vi "GetSpectrum_Fast_sub.vi"() -> (0 "array":i32[](array[numeric]), 1 "from GetStatus 2":T1, 2 "from Get Acq Data":u32, 3 "from Start Acq":u32)   [LabVIEW 2021]
uses:
  <userlib>/atmcd32d.llb/Error Code Enum typedef.ctl
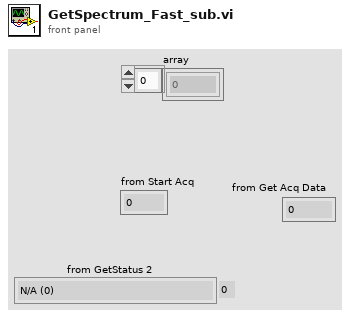
[diagram p1: front panel]
types:
  T1 = typedef "Error Code Enum typedef.ctl" = enum32{"N/A (0)", "DRV_ERROR_CODES", "DRV_SUCCESS", "DRV_VXDNOTINSTALLED", "DRV_ERROR_SCAN", "DRV_ERROR_CHECK_SUM", "DRV_ERROR_FILELOAD", "DRV_UNKNOWN_FUNC", "DRV_ERROR_VXD_INIT", "DRV_ERROR_ADDRESS", "DRV_ERROR_PAGELOCK", "DRV_ERROR_PAGEUNLOCK", "DRV_ERROR_BOARDTEST", "DRV_ERROR_ACK", "DRV_ERROR_UP_FIFO", "DRV_ERROR_PATTERN", "N/A (16)", "DRV_ACQUISITION_ERRORS", "DRV_ACQ_BUFFER", "DRV_ACQ_DOWNFIFO_FULL", "DRV_PROC_UNKONWN_INSTRUCTION", "DRV_ILLEGAL_OP_CODE", "DRV_KINETIC_TIME_NOT_MET", "DRV_ACCUM_TIME_NOT_MET", "DRV_NO_NEW_DATA", "N/A (25)", "DRV_SPOOLERROR", "N/A (27)", "N/A (28)", "N/A (29)", "N/A (30)", "N/A (31)", "N/A (32)", "DRV_TEMPERATURE_CODES", "DRV_TEMPERATURE_OFF", "DRV_TEMPERATURE_NOT_STABILIZED", "DRV_TEMPERATURE_STABILIZED", "DRV_TEMPERATURE_NOT_REACHED", "DRV_TEMPERATURE_OUT_RANGE", "DRV_TEMPERATURE_NOT_SUPPORTED", "DRV_TEMPERATURE_DRIFT", "N/A (41)", "N/A (42)", "N/A (43)", "N/A (44)", "N/A (45)", "N/A (46)", "N/A (47)", "N/A (48)", "DRV_GENERAL_ERRORS", "DRV_INVALID_AUX", "DRV_COF_NOTLOADED", "DRV_FPGAPROG", "DRV_FLEXERROR", "DRV_GPIBERROR", "N/A (55)", "N/A (56)", "N/A (57)", "N/A (58)", "N/A (59)", "N/A (60)", "N/A (61)", "N/A (62)", "N/A (63)", "DRV_DATATYPE", "DRV_DRIVER_ERRORS", "DRV_P1INVALID", "DRV_P2INVALID", "DRV_P3INVALID", "DRV_P4INVALID", "DRV_INIERROR", "DRV_COFERROR", "DRV_ACQUIRING", "DRV_IDLE", "DRV_TEMPCYCLE", "DRV_NOT_INITIALIZED", "DRV_P5INVALID", "DRV_P6INVALID", "DRV_INVALID_MODE", "DRV_INVALID_FILTER", "DRV_I2CERRORS", "DRV_I2CDEVNOTFOUND", "DRV_I2CTIMEOUT", "DRV_P7INVALID", "N/A (84)", "N/A (85)", "N/A (86)", "N/A (87)", "N/A (88)", "N/A (89)", "DRV_IOCERROR", "DRV_VRMVERSIONERROR"}
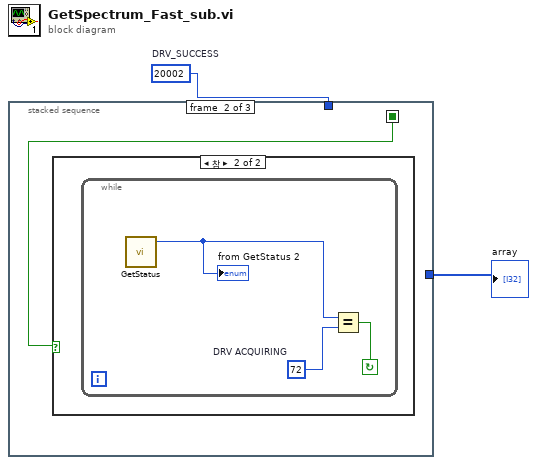
[diagram p0: block diagram]
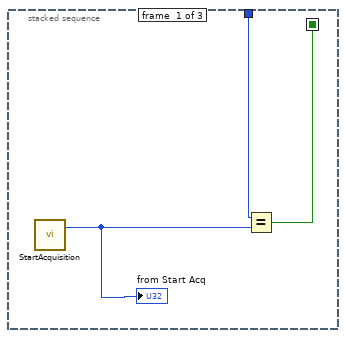
[diagram p2: hidden frame]
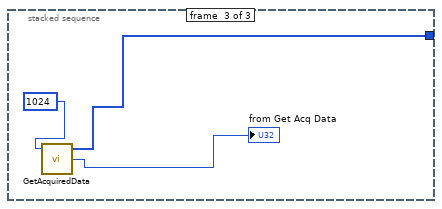
[diagram p4: hidden frame]
diagram:
  w2 = 20002  # DRV_SUCCESS
  n1 = stacked-sequence {
    seq-local: [w4 _ _] -> [_ w6 _]
    tunnel: w2 -> [w5 _ _]
    tunnel: [_ _ w10] -> w1
    frame #0 {
      n2 = call <userlib>:"StartAcquisition.vi"() -> ("DLL error code"=w3:u32)  [unwired: 2 in, 1 out]
      "from Start Acq" <- w3
      n3 = Equal?(x=w5, y=w3) -> (x = y?=w4:bool)
    }
    frame #1 {
      n4 = case shown="참" w6 {
        frame False {
        }
        frame True {
          n5 = while {
            stop <- w9 continue-if-true
            w8 = u16 72  # DRV ACQUIRING
            n6 = call <userlib>:"GetStatus.vi"() -> ("status"=w7:T1)  [unwired: 3 in, 2 out]
            "from GetStatus 2" <- w7
            n7 = Equal?(x=w7, y=w8) -> (x = y?=w9:bool)
          }
        }
      }
    }
    frame #2 {
      n8 = call <userlib>:"GetAcquiredData.vi"("size"=u32 1024) -> ("DLL error code"=→"from Get Acq Data":u32, "array"=w10:i32[])  [unwired: 2 in, 1 out]
    }
  }
  "array" <- w1
